vi "string test-1.vi"(3 "Input":dbl[](array[numeric])) -> (1 "Output in binary":i32[][](array[numeric]) format="%b", 2 "Output in Desimal":i32[][](array[numeric]))   [LabVIEW 2015]
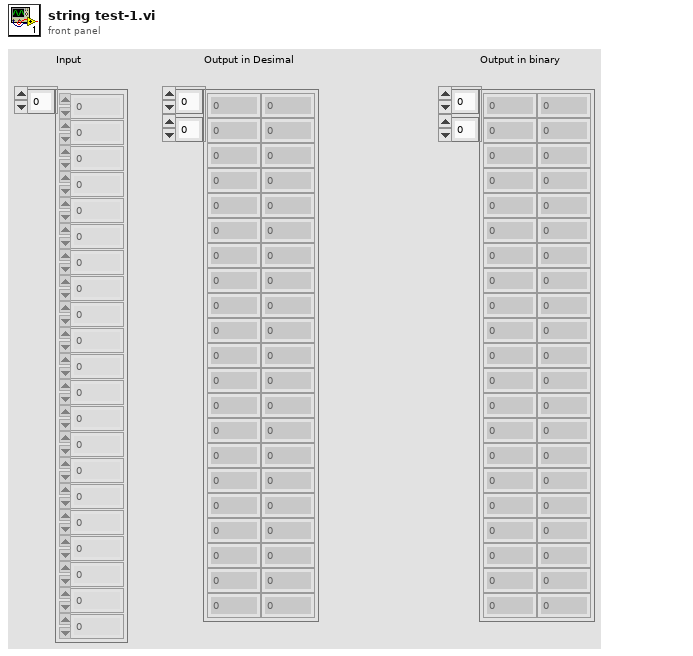
[diagram p1: front panel]
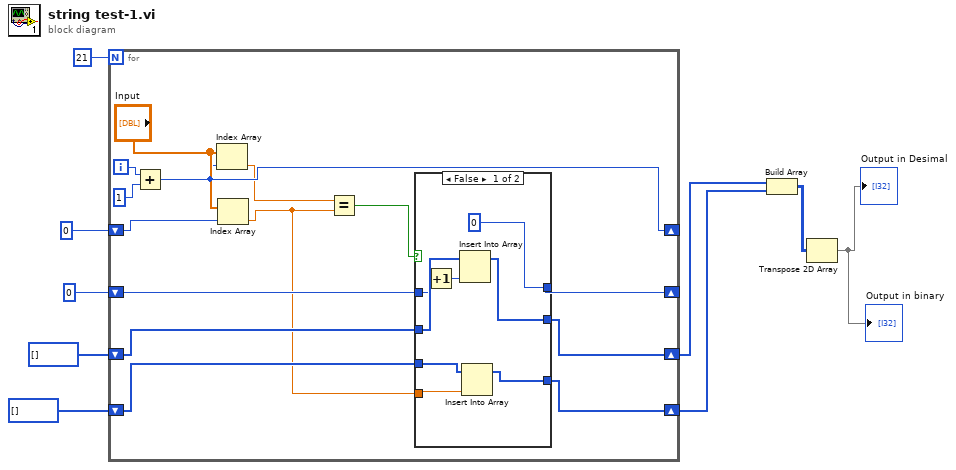
[diagram p0: block diagram]
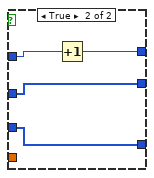
[diagram p2: hidden frame]
diagram:
  n1 = for {
    N: 21 -> [_]
    shift-right: [w13] -> w4
    shift-left: i32[] [] -> [w18]
    shift-right: [w16] -> _
    shift-left: 0 -> [w17]
    shift-right: [w15] -> _
    shift-left: 0 -> [w23]
    shift-right: [w11] -> w3
    shift-left: i32[] [] -> [w14]
    i -> [w21]
    n2 = Add(x=w21, y=1) -> (x+y=w15:i32)
    n3 = Index Array(array="Input", index=w15) -> (element=w12:dbl)
    n4 = Index Array(array="Input", index=w23) -> (element=w10:dbl)
    n5 = Equal?(x=w12, y=w10) -> (x = y?=w19:bool)
    n6 = case shown="False" w19 {
      tunnel: [w30 w34] -> w13
      tunnel: [0 w35] -> w16
      tunnel: w18 -> [w29 w34]
      tunnel: w17 -> [w28 w33]
      tunnel: w14 -> [w26 w32]
      tunnel: [w25 w32] -> w11
      tunnel: w10 -> [w24 _]
      frame False {
        n7 = Increment(x=w28) -> (x+1=w27:i32)
        n8 = Insert Into Array "Insert Into Array"(array=w29, new element=w27) -> (w30:i32[])  [unwired: 1 in]
        n9 = Insert Into Array(array=w26, new element=w24) -> (w25:i32[])  [unwired: 1 in]
      }
      frame True {
        n10 = Increment(x=w33) -> (x+1=w35:i32)
      }
    }
  }
  n11 = Build Array(w4, w3) -> (w2:i32[][])
  n12 = Transpose 2D Array(2D array=w2) -> (transposed array=→"Output in Desimal" →"Output in binary":i32[][])
